vi "PIV_Multi_Run.vi"() -> ()   [LabVIEW 2011]
panel:
  in  "PIV Process Array":T1(array[cluster])=[{"XYZ Translation"=[0.0, 0.0, 0.0], "Data Folder"=path "E:/Experiements/NACA0015_NM_C/1A/Analysis", "Output Directory"=path "T:/Ensight_Data/NACA0015/NACA0015_NM_C", "Case Name"="1A", "PIV Meas Plane"=enum."XZ", "PIV Freq (Hz)"=7.25, "Invert U"=TRUE, "Invert V"=FALSE, "Mode"=enum."Check", "Kurt Tolerance"=10.0}, {"XYZ Translation"=[0.0, 0.0, 0.0], "Data Folder"=path "E:/Experiements/NACA0015_NM_C/1B/Analysis", "Output Directory"=path "T:/Ensight_Data/NACA0015/NACA0015_NM_C", "Case Name"="1B", "PIV Meas Plane"=enum."XZ", "PIV Freq (Hz)"=7.25, "Invert U"=TRUE, "Invert V"=FALSE, "Mode"=enum."Check", "Kurt Tolerance"=10.0}, {"XYZ Translation"=[0.0, 0.0, 0.0], "Data Folder"=path "E:/Experiements/NACA0015_NM_C/1C/Analysis", "Output Directory"=path "T:/Ensight_Data/NACA0015/NACA0015_NM_C", "Case Name"="1C", "PIV Meas Plane"=enum."XZ", "PIV Freq (Hz)"=7.25, "Invert U"=TRUE, "Invert V"=FALSE, "Mode"=enum."Check", "Kurt Tolerance"=10.0}, {"XYZ Translation"=[0.0, 0.0, 0.0], "Data Folder"=path "E:/Experiements/NACA0015_NM_C/1D/Analysis", "Output Directory"=path "T:/Ensight_Data/NACA0015/NACA0015_NM_C", "Case Name"="1D", "PIV Meas Plane"=enum."XZ", "PIV Freq (Hz)"=7.25, "Invert U"=TRUE, "Invert V"=FALSE, "Mode"=enum."Check", "Kurt Tolerance"=10.0}, {"XYZ Translation"=[0.0, 0.0, 0.0], "Data Folder"=path "E:/Experiements/NACA0015_NM_C/1E/Analysis", "Output Directory"=path "T:/Ensight_Data/NACA0015/NACA0015_NM_C", "Case Name"="1E", "PIV Meas Plane"=enum."XZ", "PIV Freq (Hz)"=7.25, "Invert U"=TRUE, "Invert V"=FALSE, "Mode"=enum."Check", "Kurt Tolerance"=10.0}, {"XYZ Translation"=[0.0, 0.0, 0.0], "Data Folder"=path "E:/Experiements/NACA0015_NM_C/1F/Analysis", "Output Directory"=path "T:/Ensight_Data/NACA0015/NACA0015_NM_C", "Case Name"="1F", "PIV Meas Plane"=enum."XZ", "PIV Freq (Hz)"=7.25, "Invert U"=TRUE, "Invert V"=FALSE, "Mode"=enum."Check", "Kurt Tolerance"=10.0}, {"XYZ Translation"=[0.0, 0.0, 0.0], "Data Folder"=path "E:/Experiements/NACA0015_NM_C/1G/Analysis", "Output Directory"=path "T:/Ensight_Data/NACA0015/NACA0015_NM_C", "Case Name"="1G", "PIV Meas Plane"=enum."XZ", "PIV Freq (Hz)"=7.25, "Invert U"=TRUE, "Invert V"=FALSE, "Mode"=enum."Check", "Kurt Tolerance"=10.0}, {"XYZ Translation"=[0.0, 0.0, 0.0], "Data Folder"=path "E:/Experiements/NACA0015_NM_C/1H/Analysis", "Output Directory"=path "T:/Ensight_Data/NACA0015/NACA0015_NM_C", "Case Name"="1H", "PIV Meas Plane"=enum."XZ", "PIV Freq (Hz)"=7.25, "Invert U"=TRUE, "Invert V"=FALSE, "Mode"=enum."Check", "Kurt Tolerance"=10.0}, {"XYZ Translation"=[0.0, 0.0, 0.0], "Data Folder"=path "E:/Experiements/NACA0015_NM_C/1I/Analysis", "Output Directory"=path "T:/Ensight_Data/NACA0015/NACA0015_NM_C", "Case Name"="1I", "PIV Meas Plane"=enum."XZ", "PIV Freq (Hz)"=7.25, "Invert U"=TRUE, "Invert V"=FALSE, "Mode"=enum."Check", "Kurt Tolerance"=10.0}, {"XYZ Translation"=[0.0, 0.0, 0.0], "Data Folder"=path "E:/Experiements/NACA0015_NM_C/1J/Analysis", "Output Directory"=path "T:/Ensight_Data/NACA0015/NACA0015_NM_C", "Case Name"="1J", "PIV Meas Plane"=enum."XZ", "PIV Freq (Hz)"=7.25, "Invert U"=TRUE, "Invert V"=FALSE, "Mode"=enum."Check", "Kurt Tolerance"=10.0}, {"XYZ Translation"=[0.0, 0.0, 0.0], "Data Folder"=path "E:/Experiements/NACA0015_NM_C/1K/Analysis", "Output Directory"=path "T:/Ensight_Data/NACA0015/NACA0015_NM_C", "Case Name"="1K", "PIV Meas Plane"=enum."XZ", "PIV Freq (Hz)"=7.25, "Invert U"=TRUE, "Invert V"=FALSE, "Mode"=enum."Check", "Kurt Tolerance"=10.0}, {"XYZ Translation"=[0.0, 0.0, 0.0], "Data Folder"=path "E:/Experiements/NACA0015_NM_C/1L/Analysis", "Output Directory"=path "T:/Ensight_Data/NACA0015/NACA0015_NM_C", "Case Name"="1L", "PIV Meas Plane"=enum."XZ", "PIV Freq (Hz)"=7.25, "Invert U"=TRUE, "Invert V"=FALSE, "Mode"=enum."Check", "Kurt Tolerance"=10.0}, {"XYZ Translation"=[0.0, 0.0, 0.0], "Data Folder"=path "E:/Experiements/NACA0015_NM_C/2A/Analysis", "Output Directory"=path "T:/Ensight_Data/NACA0015/NACA0015_NM_C", "Case Name"="2A", "PIV Meas Plane"=enum."XZ", "PIV Freq (Hz)"=7.25, "Invert U"=TRUE, "Invert V"=FALSE, "Mode"=enum."Check", "Kurt Tolerance"=10.0}, {"XYZ Translation"=[0.0, 0.0, 0.0], "Data Folder"=path "E:/Experiements/NACA0015_NM_C/2B/Analysis", "Output Directory"=path "T:/Ensight_Data/NACA0015/NACA0015_NM_C", "Case Name"="2B", "PIV Meas Plane"=enum."XZ", "PIV Freq (Hz)"=7.25, "Invert U"=TRUE, "Invert V"=FALSE, "Mode"=enum."Check", "Kurt Tolerance"=10.0}, {"XYZ Translation"=[0.0, 0.0, 0.0], "Data Folder"=path "E:/Experiements/NACA0015_NM_C/2C/Analysis", "Output Directory"=path "T:/Ensight_Data/NACA0015/NACA0015_NM_C", "Case Name"="2C", "PIV Meas Plane"=enum."XZ", "PIV Freq (Hz)"=7.25, "Invert U"=TRUE, "Invert V"=FALSE, "Mode"=enum."Check", "Kurt Tolerance"=10.0}, {"XYZ Translation"=[0.0, 0.0, 0.0], "Data Folder"=path "E:/Experiements/NACA0015_NM_C/2D/Analysis", "Output Directory"=path "T:/Ensight_Data/NACA0015/NACA0015_NM_C", "Case Name"="2D", "PIV Meas Plane"=enum."XZ", "PIV Freq (Hz)"=7.25, "Invert U"=TRUE, "Invert V"=FALSE, "Mode"=enum."Check", "Kurt Tolerance"=10.0}, {"XYZ Translation"=[0.0, 0.0, 0.0], "Data Folder"=path "E:/Experiements/NACA0015_NM_C/2E/Analysis", "Output Directory"=path "T:/Ensight_Data/NACA0015/NACA0015_NM_C", "Case Name"="2E", "PIV Meas Plane"=enum."XZ", "PIV Freq (Hz)"=7.25, "Invert U"=TRUE, "Invert V"=FALSE, "Mode"=enum."Check", "Kurt Tolerance"=10.0}, {"XYZ Translation"=[0.0, 0.0, 0.0], "Data Folder"=path "E:/Experiements/NACA0015_NM_C/2F/Analysis", "Output Directory"=path "T:/Ensight_Data/NACA0015/NACA0015_NM_C", "Case Name"="2F", "PIV Meas Plane"=enum."XZ", "PIV Freq (Hz)"=7.25, "Invert U"=TRUE, "Invert V"=FALSE, "Mode"=enum."Check", "Kurt Tolerance"=10.0}, {"XYZ Translation"=[0.0, 0.0, 0.0], "Data Folder"=path "E:/Experiements/NACA0015_NM_C/2G/Analysis", "Output Directory"=path "T:/Ensight_Data/NACA0015/NACA0015_NM_C", "Case Name"="2G", "PIV Meas Plane"=enum."XZ", "PIV Freq (Hz)"=7.25, "Invert U"=TRUE, "Invert V"=FALSE, "Mode"=enum."Check", "Kurt Tolerance"=10.0}, {"XYZ Translation"=[0.0, 0.0, 0.0], "Data Folder"=path "E:/Experiements/NACA0015_NM_C/2H/Analysis", "Output Directory"=path "T:/Ensight_Data/NACA0015/NACA0015_NM_C", "Case Name"="2H", "PIV Meas Plane"=enum."XZ", "PIV Freq (Hz)"=7.25, "Invert U"=TRUE, "Invert V"=FALSE, "Mode"=enum."Check", "Kurt Tolerance"=10.0}, {"XYZ Translation"=[0.0, 0.0, 0.0], "Data Folder"=path "E:/Experiements/NACA0015_NM_C/2I/Analysis", "Output Directory"=path "T:/Ensight_Data/NACA0015/NACA0015_NM_C", "Case Name"="2I", "PIV Meas Plane"=enum."XZ", "PIV Freq (Hz)"=7.25, "Invert U"=TRUE, "Invert V"=FALSE, "Mode"=enum."Check", "Kurt Tolerance"=10.0}, {"XYZ Translation"=[0.0, 0.0, 0.0], "Data Folder"=path "E:/Experiements/NACA0015_NM_C/2J/Analysis", "Output Directory"=path "T:/Ensight_Data/NACA0015/NACA0015_NM_C", "Case Name"="2J", "PIV Meas Plane"=enum."XZ", "PIV Freq (Hz)"=7.25, "Invert U"=TRUE, "Invert V"=FALSE, "Mode"=enum."Check", "Kurt Tolerance"=10.0}, {"XYZ Translation"=[0.0, 0.0, 0.0], "Data Folder"=path "E:/Experiements/NACA0015_NM_C/2K/Analysis", "Output Directory"=path "T:/Ensight_Data/NACA0015/NACA0015_NM_C", "Case Name"="2K", "PIV Meas Plane"=enum."XZ", "PIV Freq (Hz)"=7.25, "Invert U"=TRUE, "Invert V"=FALSE, "Mode"=enum."Check", "Kurt Tolerance"=10.0}, {"XYZ Translation"=[0.0, 0.0, 0.0], "Data Folder"=path "E:/Experiements/NACA0015_NM_C/2L/Analysis", "Output Directory"=path "T:/Ensight_Data/NACA0015/NACA0015_NM_C", "Case Name"="2L", "PIV Meas Plane"=enum."XZ", "PIV Freq (Hz)"=7.25, "Invert U"=TRUE, "Invert V"=FALSE, "Mode"=enum."Check", "Kurt Tolerance"=10.0}, {"XYZ Translation"=[0.0, 0.0, 0.0], "Data Folder"=path "E:/Experiements/NACA0015_NM_C/3B/Analysis", "Output Directory"=path "T:/Ensight_Data/NACA0015/NACA0015_NM_C", "Case Name"="3B", "PIV Meas Plane"=enum."XZ", "PIV Freq (Hz)"=7.25, "Invert U"=TRUE, "Invert V"=FALSE, "Mode"=enum."Check", "Kurt Tolerance"=10.0}, {"XYZ Translation"=[0.0, 0.0, 0.0], "Data Folder"=path "E:/Experiements/NACA0015_NM_C/4B/Analysis", "Output Directory"=path "T:/Ensight_Data/NACA0015/NACA0015_NM_C", "Case Name"="4B", "PIV Meas Plane"=enum."XZ", "PIV Freq (Hz)"=7.25, "Invert U"=TRUE, "Invert V"=FALSE, "Mode"=enum."Check", "Kurt Tolerance"=10.0}, {"XYZ Translation"=[0.0, 0.0, 0.0], "Data Folder"=path "E:/Experiements/NACA0015_NM_C/3F/Analysis", "Output Directory"=path "T:/Ensight_Data/NACA0015/NACA0015_NM_C", "Case Name"="3F", "PIV Meas Plane"=enum."XZ", "PIV Freq (Hz)"=7.25, "Invert U"=TRUE, "Invert V"=FALSE, "Mode"=enum."Check", "Kurt Tolerance"=10.0}, {"XYZ Translation"=[0.0, 0.0, 0.0], "Data Folder"=path "E:/Experiements/NACA0015_NM_C/4F/Analysis", "Output Directory"=path "T:/Ensight_Data/NACA0015/NACA0015_NM_C", "Case Name"="4F", "PIV Meas Plane"=enum."XZ", "PIV Freq (Hz)"=7.25, "Invert U"=TRUE, "Invert V"=FALSE, "Mode"=enum."Check", "Kurt Tolerance"=10.0}, {"XYZ Translation"=[0.0, 0.0, 0.0], "Data Folder"=path "E:/Experiements/NACA0015_NM_C/3J/Analysis", "Output Directory"=path "T:/Ensight_Data/NACA0015/NACA0015_NM_C", "Case Name"="3J", "PIV Meas Plane"=enum."XZ", "PIV Freq (Hz)"=7.25, "Invert U"=TRUE, "Invert V"=FALSE, "Mode"=enum."Check", "Kurt Tolerance"=10.0}, {"XYZ Translation"=[0.0, 0.0, 0.0], "Data Folder"=path "E:/Experiements/NACA0015_NM_C/4J/Analysis", "Output Directory"=path "T:/Ensight_Data/NACA0015/NACA0015_NM_C", "Case Name"="4J", "PIV Meas Plane"=enum."XZ", "PIV Freq (Hz)"=7.25, "Invert U"=TRUE, "Invert V"=FALSE, "Mode"=enum."Check", "Kurt Tolerance"=10.0}]
  in  "Stop Button":bool
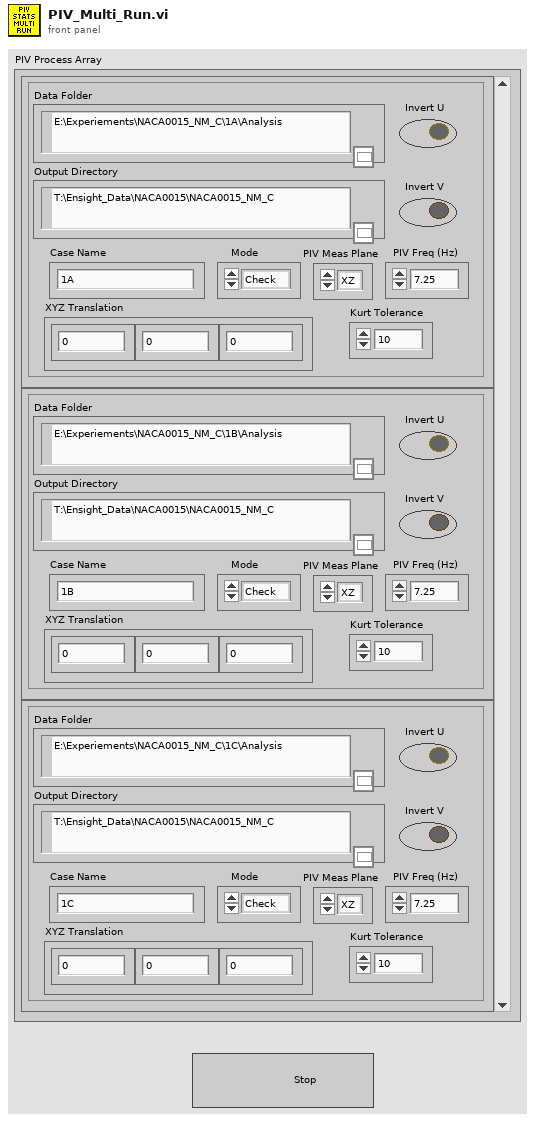
[diagram p1: front panel]
types:
  T1 = cluster{"XYZ Translation":dbl[], "Data Folder":path, "Output Directory":path, "Case Name":string, "PIV Meas Plane":enum16{"XY", "YZ", "XZ"}, "PIV Freq (Hz)":dbl, "Invert U":bool, "Invert V":bool, "Mode":enum16{"Check", "Fast", "Single", "Trans"}, "Kurt Tolerance":dbl}[]
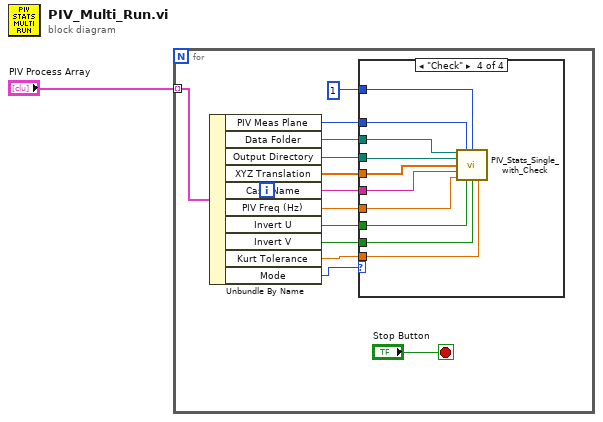
[diagram p0: block diagram]
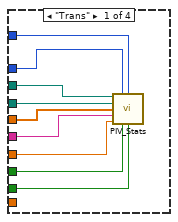
[diagram p2: hidden frame]
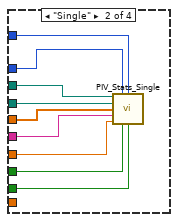
[diagram p3: hidden frame]
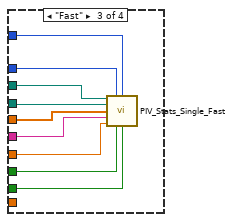
[diagram p4: hidden frame]
diagram:
  n1 = for {
    tunnel: "PIV Process Array" -> [w13] mode=indexing
    stop <- "Stop Button" stop-if-true
    n2 = Unbundle By Name(w13) -> ("PIV Meas Plane"=w10:enum16{"XY", "YZ", "XZ"}, "Data Folder"=w12:path, "Output Directory"=w11:path, "XYZ Translation"=w9:dbl[], "Case Name"=w8:string, "PIV Freq (Hz)"=w7:dbl, "Invert U"=w6:bool, "Invert V"=w5:bool, "Kurt Tolerance"=w2:dbl, "Mode"=w3:enum16{"Check", "Fast", "Single", "Trans"})
    n3 = case shown="\"Check\"" w3 {
      tunnel: w12 -> [w23 w32 w39 w49]
      tunnel: w11 -> [w22 w31 w38 w48]
      tunnel: w10 -> [w21 w30 w41 w51]
      tunnel: w9 -> [w20 w29 w37 w47]
      tunnel: w8 -> [w19 w28 w36 w46]
      tunnel: w7 -> [w18 w27 w35 w45]
      tunnel: w6 -> [w17 w26 w34 w44]
      tunnel: w5 -> [w16 w25 w33 w43]
      tunnel: 1 ("Row number") -> [w15 w24 w40 w50]
      tunnel: w2 -> [_ _ _ w42]
      frame "Trans" {
        n4 = call "PIV_Stats.vi"("Data Folder"=w23, "PIV Meas Plane"=w21, "Row number"=w15, "Output Directory"=w22, "XYZ Translation"=w20, "Case Name"=w19, "PIV Freq (Hz)"=w18, "Invert U"=w17, "Invert V"=w16) -> ()  [unwired: 3 in, 4 out]
      }
      frame "Single" {
        n5 = call "PIV_Stats_Single.vi"("Data Folder"=w32, "PIV Meas Plane"=w30, "Row number"=w24, "Output Directory"=w31, "XYZ Translation"=w29, "Case Name"=w28, "PIV Freq (Hz)"=w27, "Invert U"=w26, "Invert V"=w25) -> ()  [unwired: 4 in, 3 out]
      }
      frame "Fast" {
        n6 = call "PIV_Stats_Single_Fast.vi"("Data Folder"=w39, "PIV Meas Plane"=w41, "Row number"=w40, "Output Directory"=w38, "XYZ Translation"=w37, "Case Name"=w36, "PIV Freq (Hz)"=w35, "Invert U"=w34, "Invert V"=w33) -> ()  [unwired: 4 in, 3 out]
      }
      frame "Check" {
        n7 = call "PIV_Stats_Single_with_Check.vi"("Data Folder"=w49, "PIV Meas Plane"=w51, "Row number"=w50, "Output Directory"=w48, "XYZ Translation"=w47, "Case Name"=w46, "PIV Freq (Hz)"=w45, "Invert U"=w44, "Invert V"=w43, "Kurt Tolerance"=w42) -> ()  [unwired: 3 in, 3 out]
      }
    }
  }
